vi "Unitary_Test_Close.vi"() -> (0 "Test_passed":bool)   [LabVIEW 2015]
panel:
  out "error2 must FAIL":errorcluster
  out "error1 must be OK":errorcluster
  in  "Experience ID1":string="TestOK"
  out "Test_OK":bool[](array[boolean])=[TRUE]
  # "Test basic methods with some testing plant"
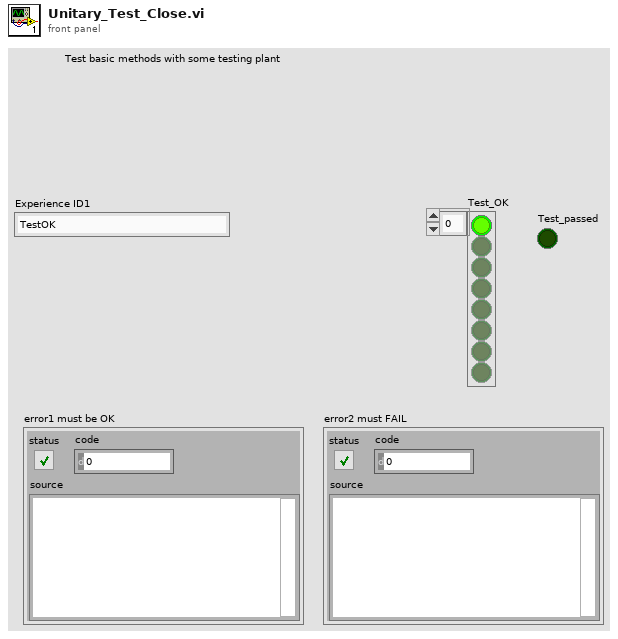
[diagram p1: front panel]
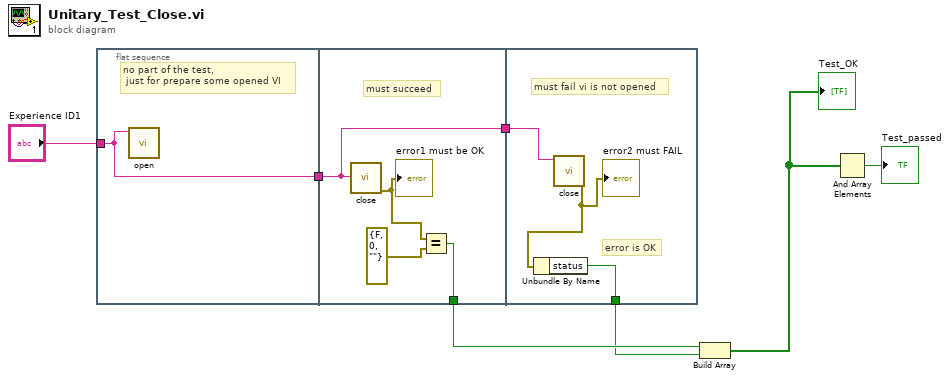
[diagram p0: block diagram]
diagram:
  n1 = flat-sequence {
    tunnel: "Experience ID1" -> [w8]
    tunnel: [w8] -> w5
    tunnel: w5 -> [w10]
    tunnel: [w10] -> w3
    tunnel: [w9] -> w2
    tunnel: w3 -> [w15]
    tunnel: [w13] -> w1
    frame #0 {
      # "no part of the test,\n just for prepare some opened VI"
      n2 = call "open.vi"("Experience ID"=w8) -> ()  [unwired: 8 in, 3 out]
    }
    frame #1 {
      # "must succeed"
      n3 = call "close.vi"("Experience ID"=w10) -> ("error out"=w12:errorcluster)  [unwired: 10 in]
      "error1 must be OK" <- w12
      n4 = Equal?(x=w12, y=errorcluster {"status"=FALSE, "code"=0, "source"=""} ("error out")) -> (x = y?=w9:bool)
    }
    frame #2 {
      # "error is OK"
      # "must fail vi is not opened"
      n5 = call "close.vi"("Experience ID"=w15) -> ("error out"=w14:errorcluster)  [unwired: 10 in]
      "error2 must FAIL" <- w14
      n6 = Unbundle By Name(w14) -> ("status"=w13:bool)
    }
  }
  n7 = Build Array(w2, w1) -> (w4:bool[])
  "Test_OK" <- w4
  n8 = And Array Elements(Boolean array=w4) -> (logical AND=→"Test_passed":bool)
